vi "wfm_feature init_mark_plot.vi"(8 "error in (no error)":errorcluster, 10 "mouse down pos":cluster{"X":dbl, "Y":dbl}, 11 "wfm_feature in":refnum<class "wfm_feature.lvclass">) -> (0 "error out":errorcluster, 3 "wfm_feature out":refnum<class "wfm_feature.lvclass">)   [LabVIEW 2018, in "wfm_feature.lvclass"]
uses:
  wfm_feature.lvclass
  subVI/mouse_state.ctl
  wfm_feature.lvclass/wfm_feature.ctl
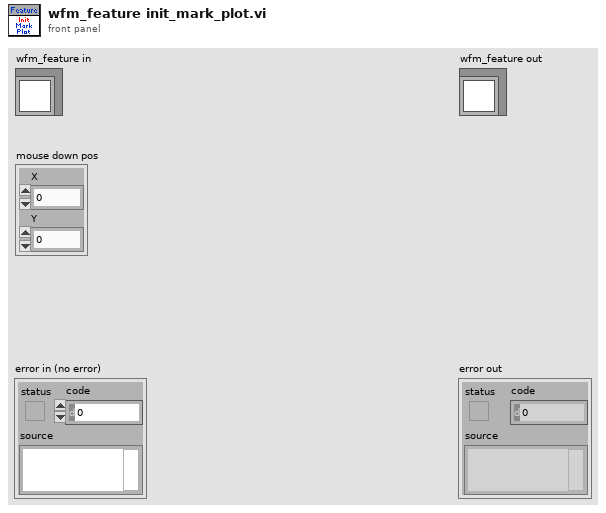
[diagram p1: front panel]
types:
  T1 = typedef "mouse_state.ctl" = enum16{"normal", "mouse down", "calc"}
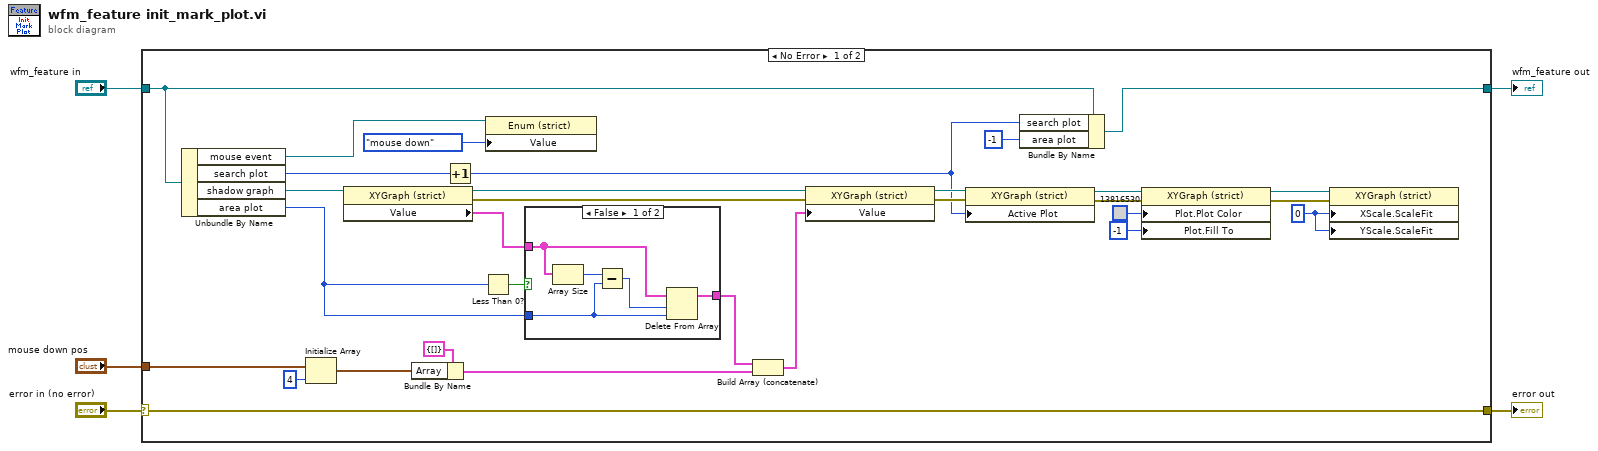
[diagram p0: block diagram]
diagram:
  n1 = case shown="No Error" "error in (no error)" {
    selector: "error in (no error)" -> [w35 w43]
    tunnel: [w35 w43] -> w4
    tunnel: [w7 w42] -> w2
    tunnel: "wfm_feature in" -> [w10 w42]
    tunnel: "mouse down pos" -> [w19 _]
    frame No Error {
      w23 = u8 0 ("X Scale.Scale Fit")
      n2 = Unbundle By Name(w10) -> ("mouse event"=w26:refnum<vi>, "search plot"=w20:i32, "shadow graph"=w21:refnum<vi>, "area plot"=w12:i32)
      n3 = Initialize Array(w19, 4 ("dimension size")) -> (w16:cluster{"X":dbl, "Y":dbl}[])
      n4 = property class="XYGraph (strict)"(reference=w21) -> (reference out=w34:refnum<vi>, error out=w33:errorcluster, "Value"=w13:cluster{"Array":cluster{"X":dbl, "Y":dbl}[]}[])  [unwired: 1 in]
      n5 = Bundle By Name(cluster=cluster{"Array":cluster{"X":dbl, "Y":dbl}[]} {"Array"=[]} ("element"), "Array"=w16) -> (w15:cluster{"Array":cluster{"X":dbl, "Y":dbl}[]})
      n6 = Increment(x=w20) -> (x+1=w9:i32)
      n7 = Less Than 0?(x=w12) -> (x < 0?=w14:bool)
      n8 = property class="Enum (strict)"(reference=w26, "Value"=mouse_state."mouse down") -> ()  [unwired: 1 in, 2 out]
      n9 = case shown="False" w14 {
        tunnel: w13 -> [w39 w41]
        tunnel: [w40 w41] -> w11
        tunnel: w12 -> [w37 _]
        frame False {
          n10 = Array Size(array=w39) -> (size(s)=w38:i32)
          n11 = Subtract(x=w38, y=w37) -> (x-y=w36:i32)
          n12 = Delete From Array(array=w39, length=w36, index=w37) -> (array with subset deleted=w40:cluster{"Array":cluster{"X":dbl, "Y":dbl}[]}[])  [unwired: 1 out]
        }
        frame True {
        }
      }
      n13 = Build Array (concatenate)(w11, w15) -> (w32:cluster{"Array":cluster{"X":dbl, "Y":dbl}[]}[])
      n14 = property class="XYGraph (strict)"(reference=w34, error in=w33, "Value"=w32) -> (reference out=w31:refnum<vi>, error out=w30:errorcluster)
      n15 = property class="XYGraph (strict)"(reference=w31, error in=w30, "Active Plot"=w9) -> (reference out=w28:refnum<vi>, error out=w27:errorcluster)
      n16 = Bundle By Name(cluster=w10, "search plot"=w9, "area plot"=-1) -> (w7:refnum<class "wfm_feature.lvclass">)
      n17 = property class="XYGraph (strict)"(reference=w28, error in=w27, "Plot.Plot Color"=u32 13816530, "Plot.Fill To"=i16 -1) -> (reference out=w24:refnum<vi>, error out=w22:errorcluster)
      n18 = property class="XYGraph (strict)"(reference=w24, error in=w22, "XScale.ScaleFit"=w23, "YScale.ScaleFit"=w23) -> ()  [unwired: 2 out]
    }
    frame Error {
    }
  }
  "error out" <- w4
  "wfm_feature out" <- w2
